vi "Get Control Data.vi"(8 "Error In":errorcluster, 10 "UID":i32, 11 "Controls":variant) -> (0 "Error Out":errorcluster, 2 "Control Data":T1, 3 "Controls":variant)   [LabVIEW 2014]
uses:
  Control Info.ctl
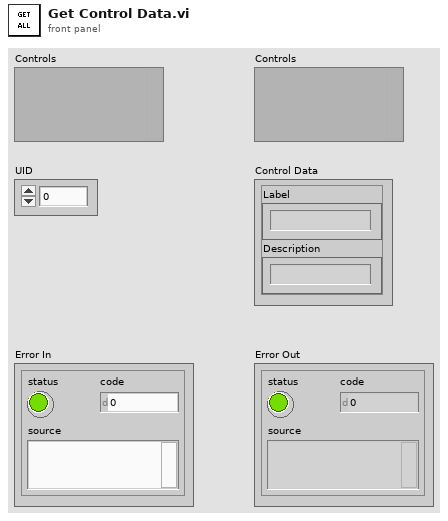
[diagram p1: front panel]
types:
  T1 = typedef "Control Info.ctl" = cluster{"Label":string, "Description":string}
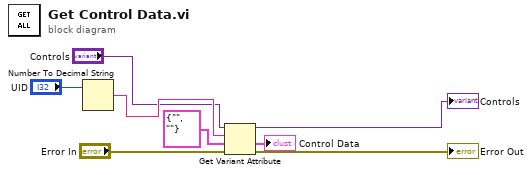
[diagram p0: block diagram]
diagram:
  n1 = Number To Decimal String(number="UID") -> (decimal integer string=w7:string)  [unwired: 1 in]
  n2 = Get Variant Attribute(Variant="Controls", name=w7, default value (empty Variant)=T1 {"Label"="", "Description"=""} ("Control Info"), error in="Error In") -> (duplicate Variant=→"Controls":variant, value=→"Control Data":T1, error out=→"Error Out":errorcluster)  [unwired: 1 out]
